vi "WinCI Compare Files.vi"(4 "version":string, 6 "compare options":T1, 7 "advanced options":variant, 8 "error in (no error)":errorcluster, 9 "compare method":T2 items=["source control provider default", "contents (silent)", "checksum (silent)", "time (silent)"], 10 "file path":path, 11 "source control reference in":T3) -> (0 "error out":errorcluster, 2 "status message":string, 3 "source control reference out":T3, 5 "file differs?":bool)   [LabVIEW 2020, in "NI_SCC_WinCI.lvlib"]
uses:
  <vilib>/SourceControl/Providers/WinCI/NI_SCC_WinCI.lvlib
  <vilib>/SourceControl/sccapi/SCCAPI Refnum.ctl
  <vilib>/SourceControl/sccapi/SCCAPI Compare Method.ctl
  <vilib>/SourceControl/sccapi/SCCAPI Compare Options.ctl
  <vilib>/SourceControl/support/SCCSup Message Strings GLBL.vi
  <vilib>/SourceControl/sccapi/NI_SCC.lvlib
panel:
  out "result":i32
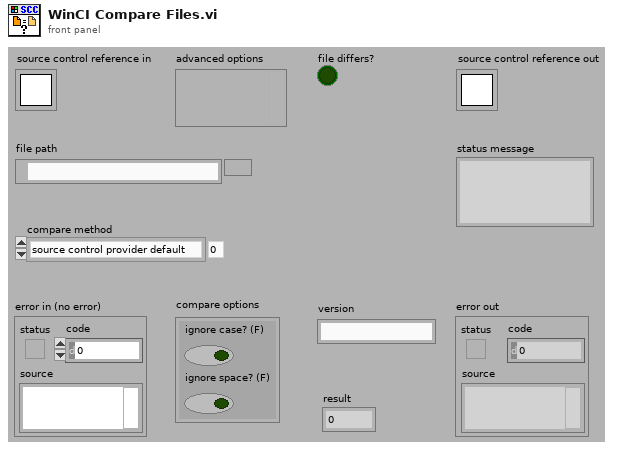
[diagram p1: front panel]
types:
  T1 = typedef "NI_SCC.lvlib/SCCAPI Compare Options.ctl" = cluster{"ignore case? (F)":bool, "ignore space? (F)":bool}
  T2 = typedef "NI_SCC.lvlib/SCCAPI Compare Method.ctl" = u16
  T3 = typedef "NI_SCC.lvlib/SCCAPI Refnum.ctl" = refnum<k1>
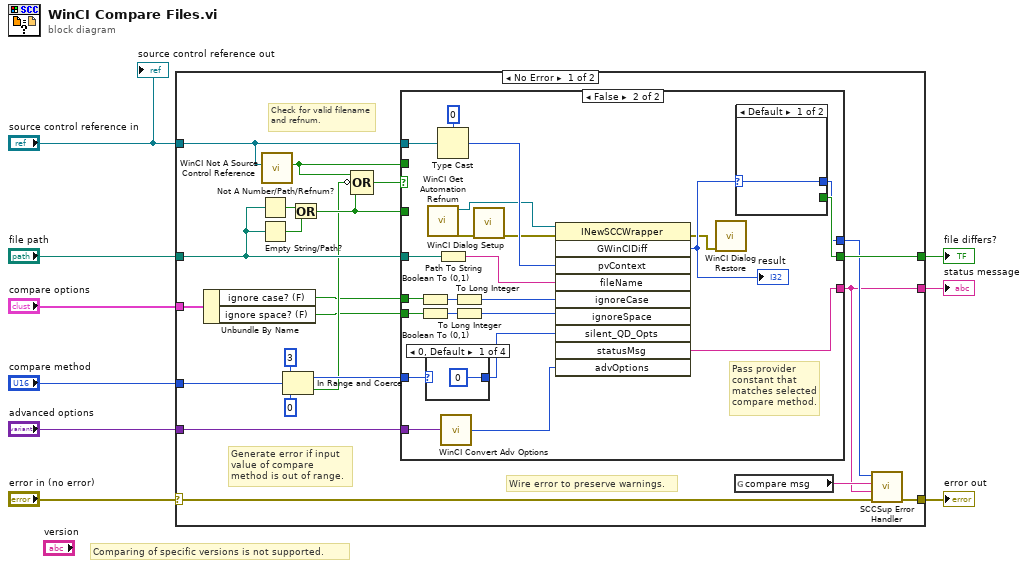
[diagram p0: block diagram]
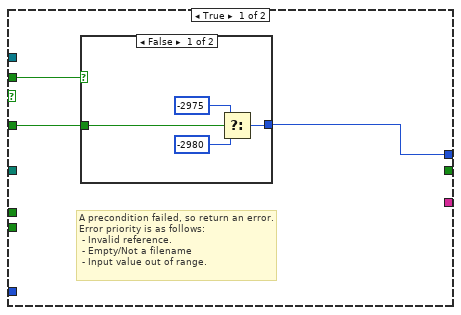
[diagram p2: hidden frame]
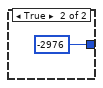
[diagram p3: hidden frame]
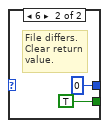
[diagram p4: hidden frame]
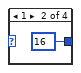
[diagram p5: hidden frame]
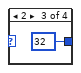
[diagram p6: hidden frame]
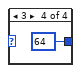
[diagram p7: hidden frame]
diagram:
  # "Comparing of specific versions is not supported."
  n1 = case shown="No Error" "error in (no error)" {
    selector: "error in (no error)" -> [w19 w70]
    tunnel: [w26 w70] -> w8
    tunnel: "source control reference in" -> [w11 _]
    tunnel: [w23 _] -> w6
    tunnel: "file path" -> [w22 _]
    tunnel: "compare method" -> [w31 _]
    tunnel: [w27 _] -> w3
    tunnel: "advanced options" -> [w18 _]
    tunnel: "compare options" -> [w14 _]
    frame No Error {
      # "Wire error to preserve warnings."
      # "Generate error if input value of compare method is out of range."
      # "Check for valid filename and refnum."
      n2 = Unbundle By Name(w14) -> ("ignore case? (F)"=w13:bool, "ignore space? (F)"=w12:bool)
      n3 = Not A Number/Path/Refnum?(number/path/refnum=w22) -> (NaN/Path/Refnum?=w21:bool)
      n4 = Empty String/Path?(string/path=w22) -> (empty?=w20:bool)
      n5 = call <vilib>:"WinCI Not A Source Control Reference.vi"("source control reference in"=w11) -> ("not a source control reference?"=w10:bool)  [unwired: 1 in, 9 out]
      n6 = In Range and Coerce(upper limit=u16 3, x=w31, lower limit=u16 0) -> (coerced(x)=w28:T2, In Range?=w15:bool)
      n7 = Or(x=w21, y=w20) -> (x .or. y?=w16:bool)
      n8 = Compound Arithmetic op=OR(w10, invert w15, w16) -> (w17:bool)
      n9 = case shown="False" w17 {
        tunnel: w11 -> [_ w62]
        tunnel: [_ w50] -> w23
        tunnel: w22 -> [_ w60]
        tunnel: w13 -> [_ w57]
        tunnel: w12 -> [_ w56]
        tunnel: w28 -> [_ w55]
        tunnel: [_ w54] -> w27
        tunnel: [w32 w53] -> w25
        tunnel: w10 -> [w34 _]
        tunnel: w18 -> [_ w52]
        tunnel: w16 -> [w33 _]
        frame True {
          # "A precondition failed, so return an error. \nError priority is as follows:\n - Invalid reference.  \n - Empty/Not a filename\n - Input value out of range."
          n10 = case shown="False" w34 {
            tunnel: w33 -> [w36 _]
            tunnel: [w35 -2976 ("result")] -> w32
            frame False {
              n11 = Select(t=-2975 ("result"), s=w36, f=-2980 ("result")) -> (s? t:f=w35:i32)
            }
            frame True {
            }
          }
        }
        frame False {
          # "Pass provider constant that matches selected compare method."
          n12 = Boolean To (0,1)(Boolean=w57) -> (0, 1=w59:i16)
          n13 = Boolean To (0,1)(Boolean=w56) -> (0, 1=w58:i16)
          n14 = case shown="0, Default" w55 {
            tunnel: [0 ("silentOptions") 16 ("silentOptions") 32 ("silentOptions") 64 ("silentOptions")] -> w48
            frame 0, Default {
            }
            frame 1 {
            }
            frame 2 {
            }
            frame 3 {
            }
          }
          n15 = call <vilib>:"WinCI Get Automation Refnum.vi"() -> ("error out"=w42:errorcluster, "automation refnum"=w43:refnum<k7>)  [unwired: 10 out]
          n16 = Type Cast(type=u32 0, x=w62) -> (*(type *) &x=w46:u32)
          n17 = Path To String(path=w60) -> (string=w47:string)
          n18 = call <vilib>:"WinCI Convert Adv Options.vi"("advanced options"=w52) -> ("command options"=w49:u32)  [unwired: 4 out]
          n19 = To Long Integer(number=w59) -> (32bit integer=w45:i32)
          n20 = To Long Integer(number=w58) -> (32bit integer=w44:i32)
          n21 = call <vilib>:"WinCI Dialog Setup.vi"("error in"=w42) -> ("error out"=w41:errorcluster)  [unwired: 10 out]
          n22 = invoke class="INewSCCWrapper" method="GWinCIDiff"(reference=w43, error in=w41, "pvContext"=w46, "fileName"=w47, "ignoreCase"=w45, "ignoreSpace"=w44, "silent_QD_Opts"=w48, "advOptions"=w49) -> (error out=w40:errorcluster, "GWinCIDiff"=w51:i32, "statusMsg"=w50:string)  [unwired: 2 in, 7 out]
          "result" <- w51
          n23 = call <vilib>:"WinCI Dialog Restore.vi"("error in"=w40) -> ()  [unwired: 11 out]
          n24 = case shown="Default" w51 {
            selector: w51 -> [w63 _]
            tunnel: [w63 0 ("result")] -> w53
            tunnel: [_ TRUE] -> w54
            frame Default {
            }
            frame 6 {
              # "File differs. Clear return value."
            }
          }
        }
      }
      n25 = global read "SCCSup Message Strings GLBL.vi" "compare msg"() -> (w24:string)
      n26 = call <vilib>:"SCCSup Error Handler.vi"("error in (no error)"=w19, "additional message"=w23, "operation message"=w24, "scc error code"=w25) -> ("error out"=w26:errorcluster)  [unwired: 7 out]
    }
    frame Error {
    }
  }
  "error out" <- w8
  "status message" <- w6
  "file differs?" <- w3
  "source control reference out" <- "source control reference in"
